vi "RoboDisplay7.vi"() -> ()   [LabVIEW 2013]
uses:
  GlobalPrevPage.vi
  GlobalPlotUpdateTime.vi
  GlobalSpeedUpdateTime.vi
  GlobalFavoriteNames.vi
  GlobalDisplayIndex.vi
  GlobalFavoritesList.vi
  GlobalRobotOffCheck.vi
  GlobalErrorCluster.vi
  GlobalErrorIndex.vi
  GlobalErrorCAN_ID.vi
  ErrorPrevValues.vi
  GlobalDataSize.vi
  GlobalSpeedArray.vi
  GlobalDataSelectArray.vi
  GlobalParamSize.vi
  GlobalFavorites.vi
  GlobalInitialParamVals.vi
  GlobalBatteryVoltageID.vi
  GlobalDataPath7.vi
  GlobalDataFileRefnum7.vi
  GlobalLabVIEWStart.vi
panel:
  out "MCU Elapsed mS 2":u32
  in  "Collect Data":bool
  out "Boolean":bool
  out "graph2labels":string[](array[string])
  out "graph1labels":string[](array[string])
  out "BATTERY VOLTAGE":dbl(knob) scale=20.0..30.0 scale format="%#_3g"
  in  "Tab Control":T1(tab)=enum."Display Data"
  out "Fav Error":bool[](array[boolean])
  in  "Remove":T2
  in  "Fav":T3
  in  "Commit":T4
  out "WAIT":bool
  in  "Reset default":bool
  out "Param #":dbl[](array[numeric])
  in  "Select 2":T5
  in  "Fav Input":dbl[](array[numeric])
  out "Value":dbl[](array[numeric])
  in  "Load":bool
  in  "Save":bool
  out "error":bool[](array[boolean])
  out "Param value":dbl[](array[numeric])
  out "Param #":dbl[](array[numeric])
  out "Param Name":string[](array[string])
  in  "Input":dbl[](array[numeric])
  in  "Page Select":dbl min=0.0 max=50.0 step=1.0
  out "Favorite Parameters":string[](array[string])
  in  "save data":bool
  in  "load data":bool
  out "Value 2":dbl[](array[numeric])
  out "Value 1":dbl[](array[numeric])
  out "Data # 2":dbl[](array[numeric])
  out "Data #":dbl[](array[numeric])
  out "Indicator":bool[](array[boolean])
  out "Array":string[](array[string])
  in  "Page":dbl min=0.0 max=50.0 step=1.0
  out "Number\nSelected":dbl
  out "Indicator 2":bool[](array[boolean])
  out "Array 2":string[](array[string])
  in  "Select":T3
  in  "?":T3
  out "Results":T6(array[cluster])
  in  "Search":string
  in  "Search \nButton":bool
  out "# of Results":i32
  in  "Speed Sel 2":enum32{"Slow", "Medium", "Fast"}[](array[radio])
  out "Speed 3":u32[](array[colorbox])
  out "Data Names 2":string[](array[string])
  out "Channel # 2":i16[](array[numeric])
  out "Data Value 2":sgl[](array[numeric]) format="%#_4g"
  out "Speed 2":u32[](array[colorbox])
  out "Data Names 1":string[](array[string])
  out "Channel # 1":i16[](array[numeric])
  out "Data Value 1":sgl[](array[numeric]) format="%#_4g"
  in  "One1":bool[](array[boolean])
  in  "One2":bool[](array[boolean])
  in  "Two1":bool[](array[boolean])
  in  "Two2":bool[](array[boolean])
  in  "Speed Sel":enum32{"Slow", "Medium", "Fast"}[](array[radio])
  in  "Clear Errors":bool
  in  "Pause Button":bool
  out "Error Description":string[](array[string])
  out "Board":string[](array[string])
  out "Error Name":string[](array[string])
  out "Freq.":dbl[](array[numeric])
  out "Time":dbl[](array[numeric])
  out "error message":bool
  out "Board Name 1":string
  out "Graph One":cluster{"Array":u32[], "Array 2":sgl[]}[](graph)
  in  "Graph\non":bool
  out "Error Name 1":string
  out "MCU Elapsed mS":u32 format="%<%H:%M:%S>t"
  in  "stop":bool
  out "Graph Two":cluster{"Array":u32[], "Array 2":sgl[]}[](graph)
  # "Robot Time:"
  # "ms timer:"
  # "DATA COLLECTION"
  # "Board"
  # "OFF"
  # "ON"
  # "Error Name"
  # "RoboDAQ\n\n(Version 7)\n\n\n\n\n\n\nCreated by: John Buzzi, Jason Cortell, Katie Hartl, Carlos Arango\n\nFall 2009"
  # "PLEASE LOOK AT SUGGESTIONS\nTAB IF YOU HAVE HELPFUL \nCOMMENTS!!"
  # "Favorites"
  # "Press [Home] to increment\nPress [End] to decrement"
  # "Press [Page Up] to increment\nPress [Page Down] to decrement"
  # "Select"
  # "Select"
  # "MAX ALLOWED: 48"
  # "NOT WORKING YET\n.\n.\n.\n.\n.\n.\n.\n......................."
  # "CAN ID"
  # "Name"
  # "Search Field"
  # "Note: Add function does not work yet"
  # "# of hits"
  # "Graphs"
  # "Graphs"
  # "Speed\n(S)   (M)   (F)"
  # "Speed\n(S)   (M)   (F)"
  # "Speed"
  # "Speed"
  # "Channel Name"
  # "One"
  # "Two"
  # "Channel Name"
  # "One"
  # "Two"
  # "SUGGESTIONS (double click text box to edit)\n\nMy to do list:\nFix error handling so that it works in the more advanced way that I had intended\nFix bug with speed select when data is de-selected and speeds are incorrect\nradio buttons\nload save data\nadd data by number\nmake index bigger\nslow default speed\n\n\nOther Suggestions/Comments (please add user input so that I can make the program better)\n- (nac) Change default folder for can_id.h and error_id.h to the Ranger Configuration folder\n\n\n\n\nNote: Strikeout = fixed"
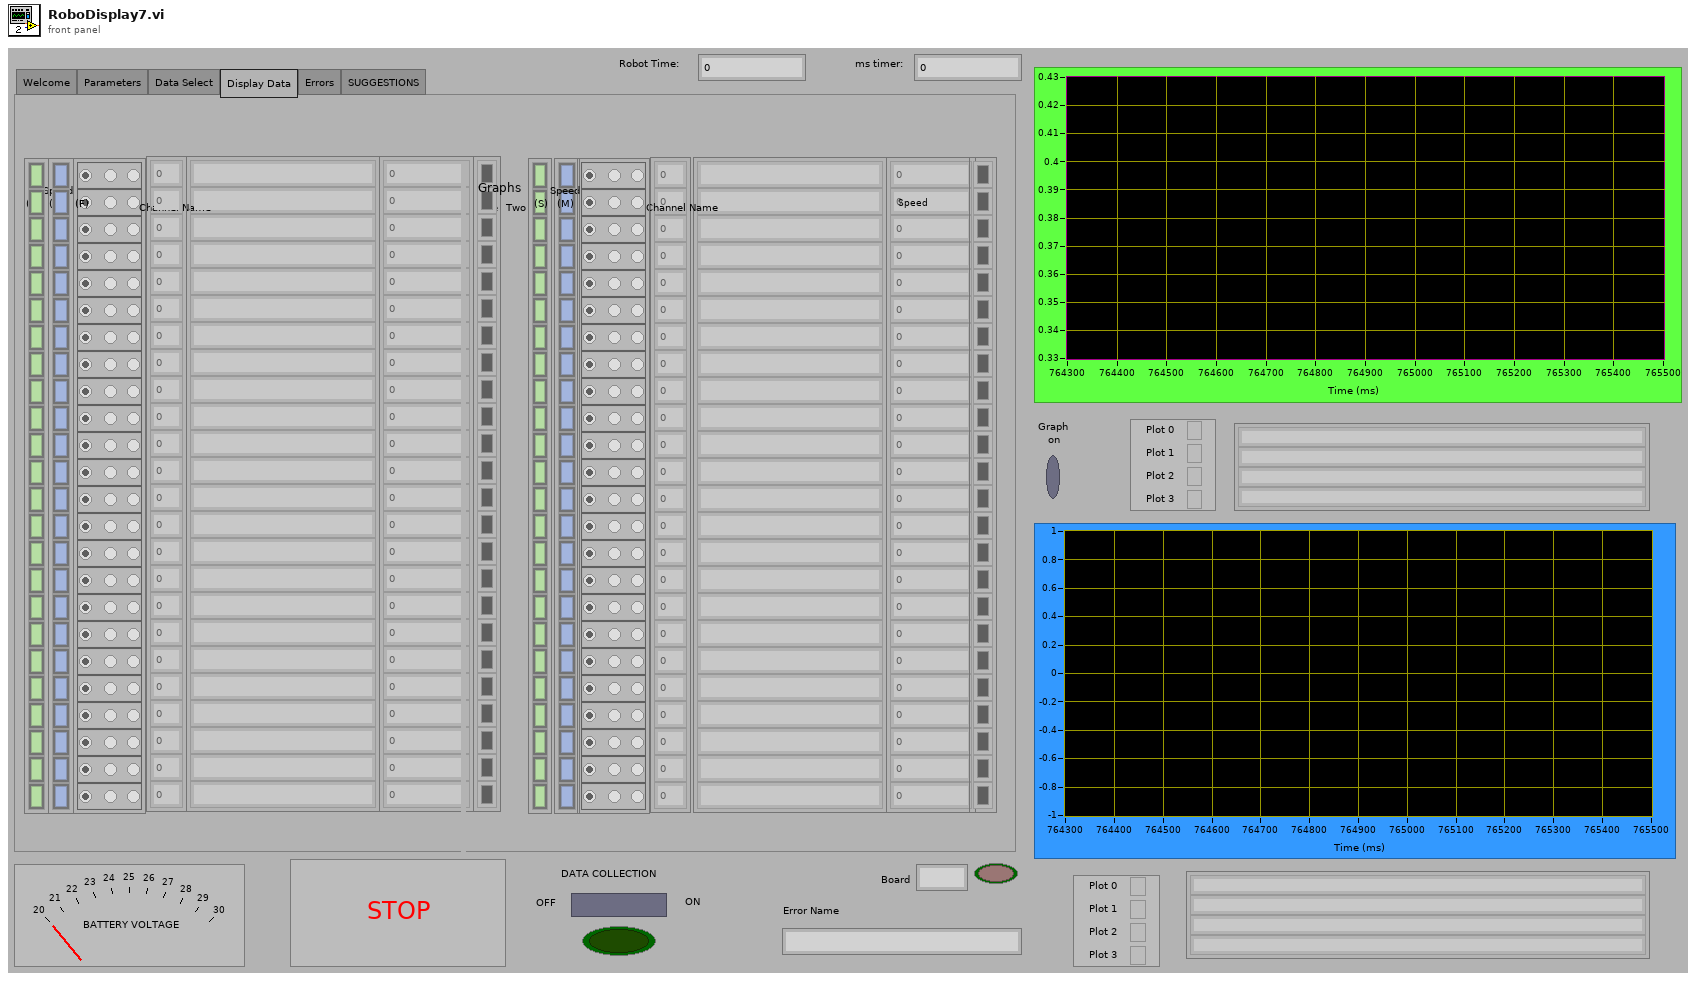
[diagram p1: front panel]
types:
  T1 = enum32{"Welcome", "Parameters", "Data Select", "Display Data", "Errors", "SUGGESTIONS"}
  T2 = cluster{"X button":bool, "X button 2":bool, "X button 3":bool, "X button 4":bool, "X button 5":bool, "X button 6":bool, "X button 7":bool, "X button 8":bool, "X button 9":bool, "X button 10":bool, "X button 11":bool, "X button 12":bool, "X button 13":bool, "X button 14":bool, "X button 15":bool, "X button 16":bool, "X button 17":bool, "X button 18":bool, "X button 19":bool, "X button 20":bool}
  T3 = cluster{"Boolean 2":bool, "Boolean 3":bool, "Boolean 4":bool, "Boolean 5":bool, "Boolean 6":bool, "Boolean 7":bool, "Boolean 8":bool, "Boolean 9":bool, "Boolean 10":bool, "Boolean 11":bool, "Boolean 12":bool, "Boolean 13":bool, "Boolean 14":bool, "Boolean 15":bool, "Boolean 16":bool, "Boolean 17":bool, "Boolean 18":bool, "Boolean 19":bool, "Boolean 20":bool, "Boolean 21":bool, "Boolean 22":bool, "Boolean 23":bool, "Boolean 24":bool, "Boolean 25":bool}
  T4 = cluster{"Boolean":bool, "Boolean 2":bool, "Boolean 3":bool, "Boolean 4":bool, "Boolean 5":bool, "Boolean 6":bool, "Boolean 7":bool, "Boolean 8":bool, "Boolean 9":bool, "Boolean 10":bool, "Boolean 11":bool, "Boolean 12":bool, "Boolean 13":bool, "Boolean 14":bool, "Boolean 15":bool, "Boolean 16":bool, "Boolean 17":bool, "Boolean 18":bool, "Boolean 19":bool, "Boolean 20":bool}
  T5 = cluster{"Boolean":bool, "Boolean 2":bool, "Boolean 3":bool, "Boolean 4":bool, "Boolean 5":bool, "Boolean 6":bool, "Boolean 7":bool, "Boolean 8":bool, "Boolean 9":bool, "Boolean 10":bool, "Boolean 11":bool, "Boolean 12":bool, "Boolean 13":bool, "Boolean 14":bool, "Boolean 15":bool, "Boolean 16":bool, "Boolean 17":bool, "Boolean 18":bool, "Boolean 19":bool, "Boolean 20":bool, "Boolean 21":bool, "Boolean 22":bool, "Boolean 23":bool, "Boolean 24":bool}
  T6 = cluster{"Result Index":dbl, "Results 3":string, "Boolean 2":bool}[]
  T7 = cluster{"Error ID":i32, "Board ID":i32, "Time":u32, "Frequency":i32}[]
  T8 = enum16{"open", "replace", "create", "open or create", "replace or create", "replace or create with confirmation"}
  T9 = cluster{"Numeric":dbl, "String":string, "ignore case? (F)":bool}
  T10 = cluster{"Numeric":dbl, "String":string, "ignore case? (F)":bool}[]
  T11 = cluster{"Frequency":dbl, "Description":string, "Error Name":string, "Board Name":string, " Board Source":dbl, "Timestamp":dbl}[]
  T12 = cluster{"Frequency":dbl, "Description":string, "Error Name":string, "Board Name":string, " Board Source":dbl, "Timestamp":dbl}
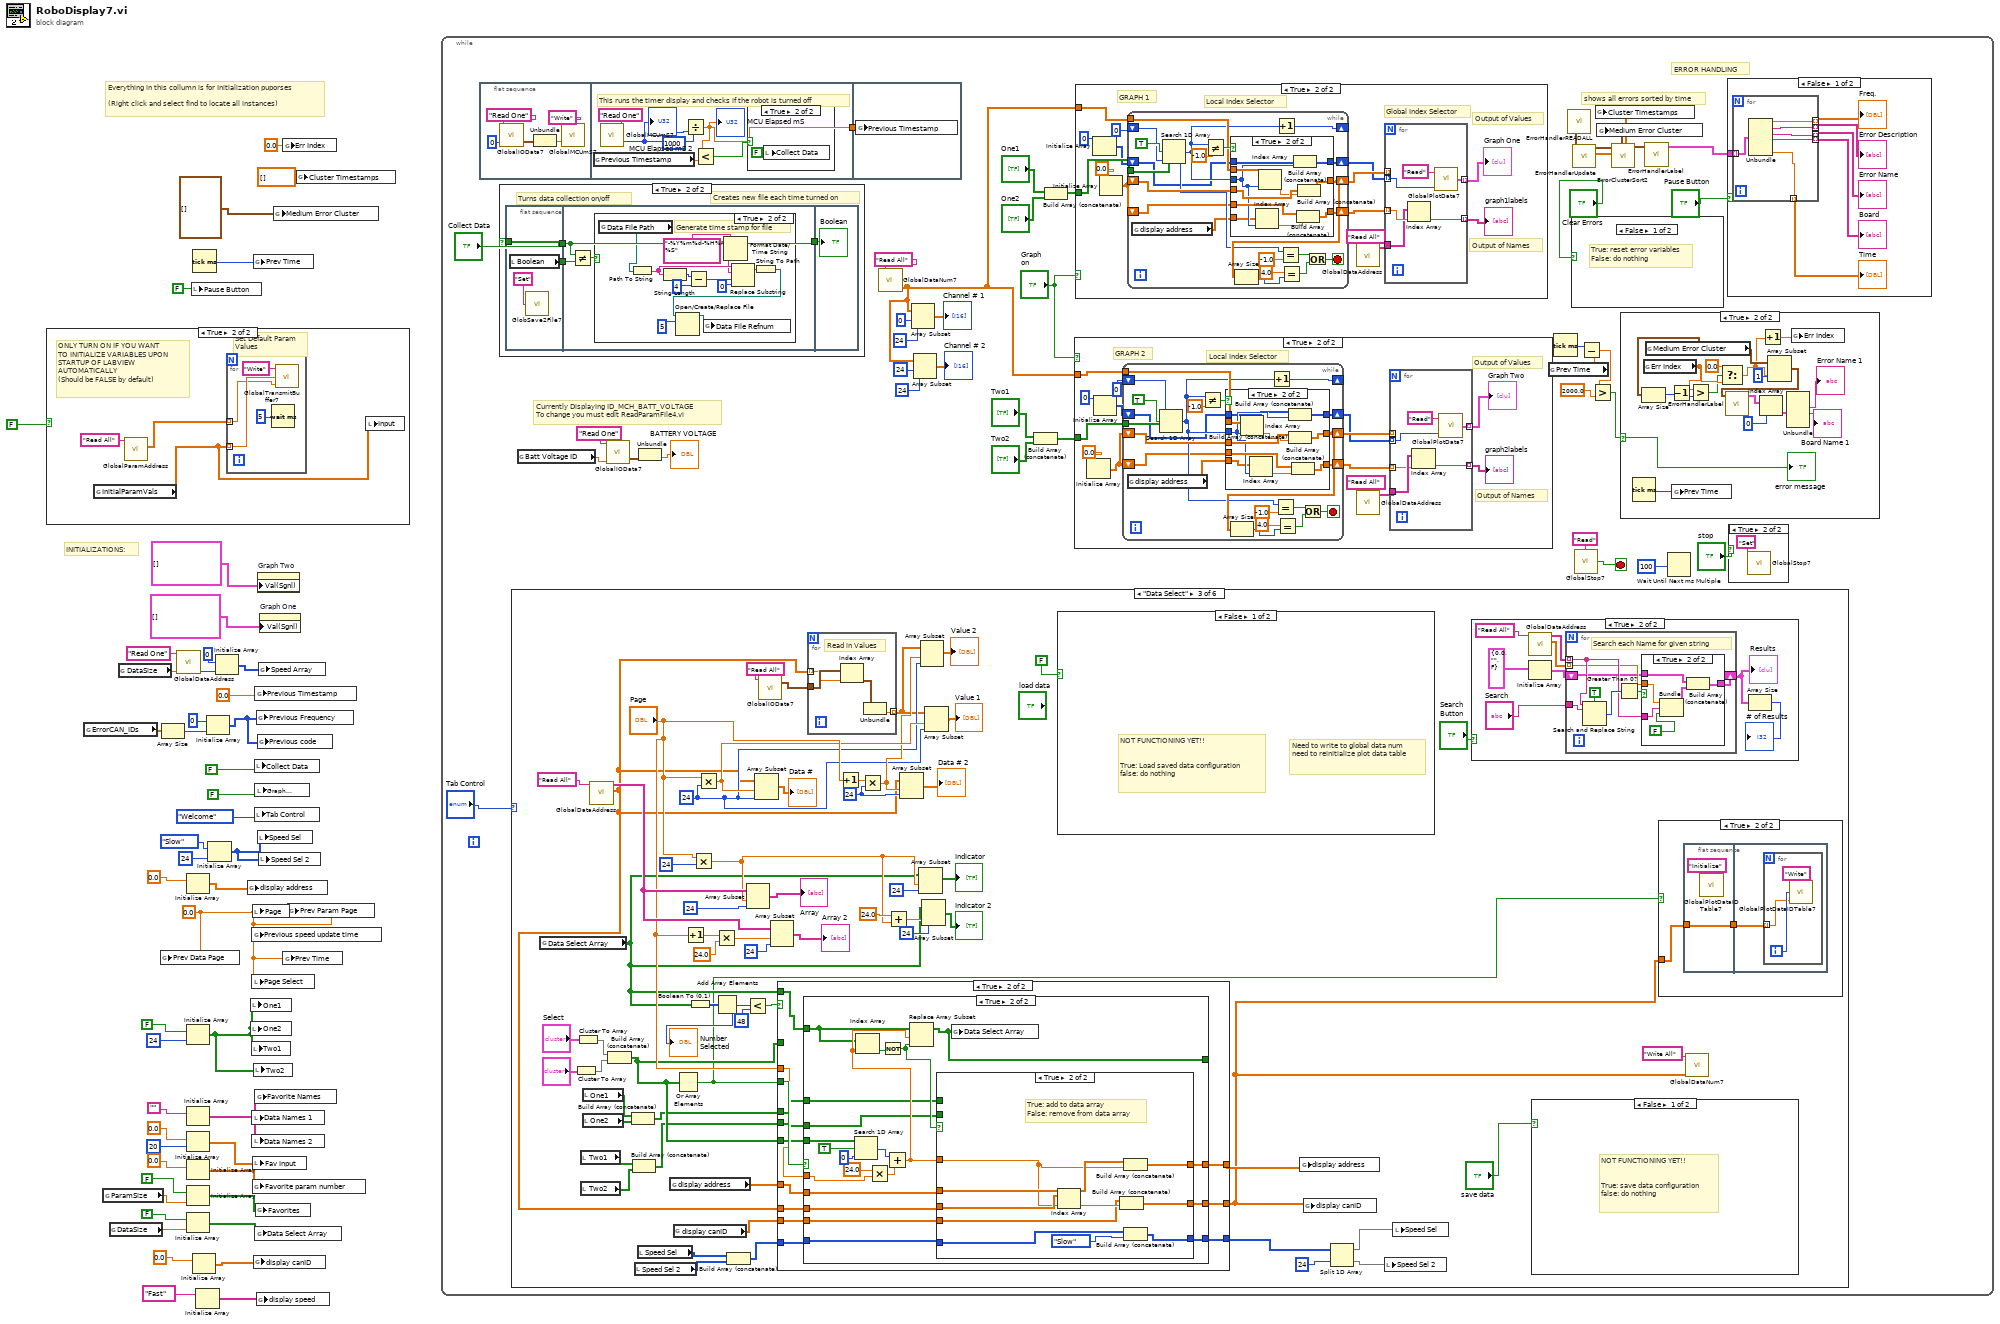
[diagram p0: block diagram]
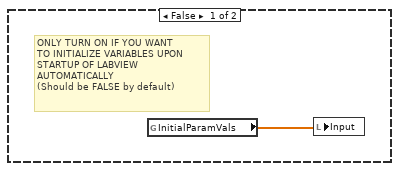
[diagram p2: hidden frame]
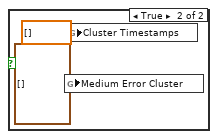
[diagram p3: hidden frame]
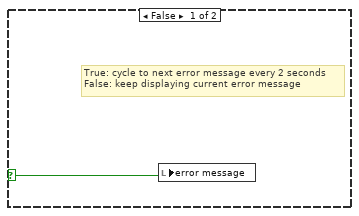
[diagram p4: hidden frame]
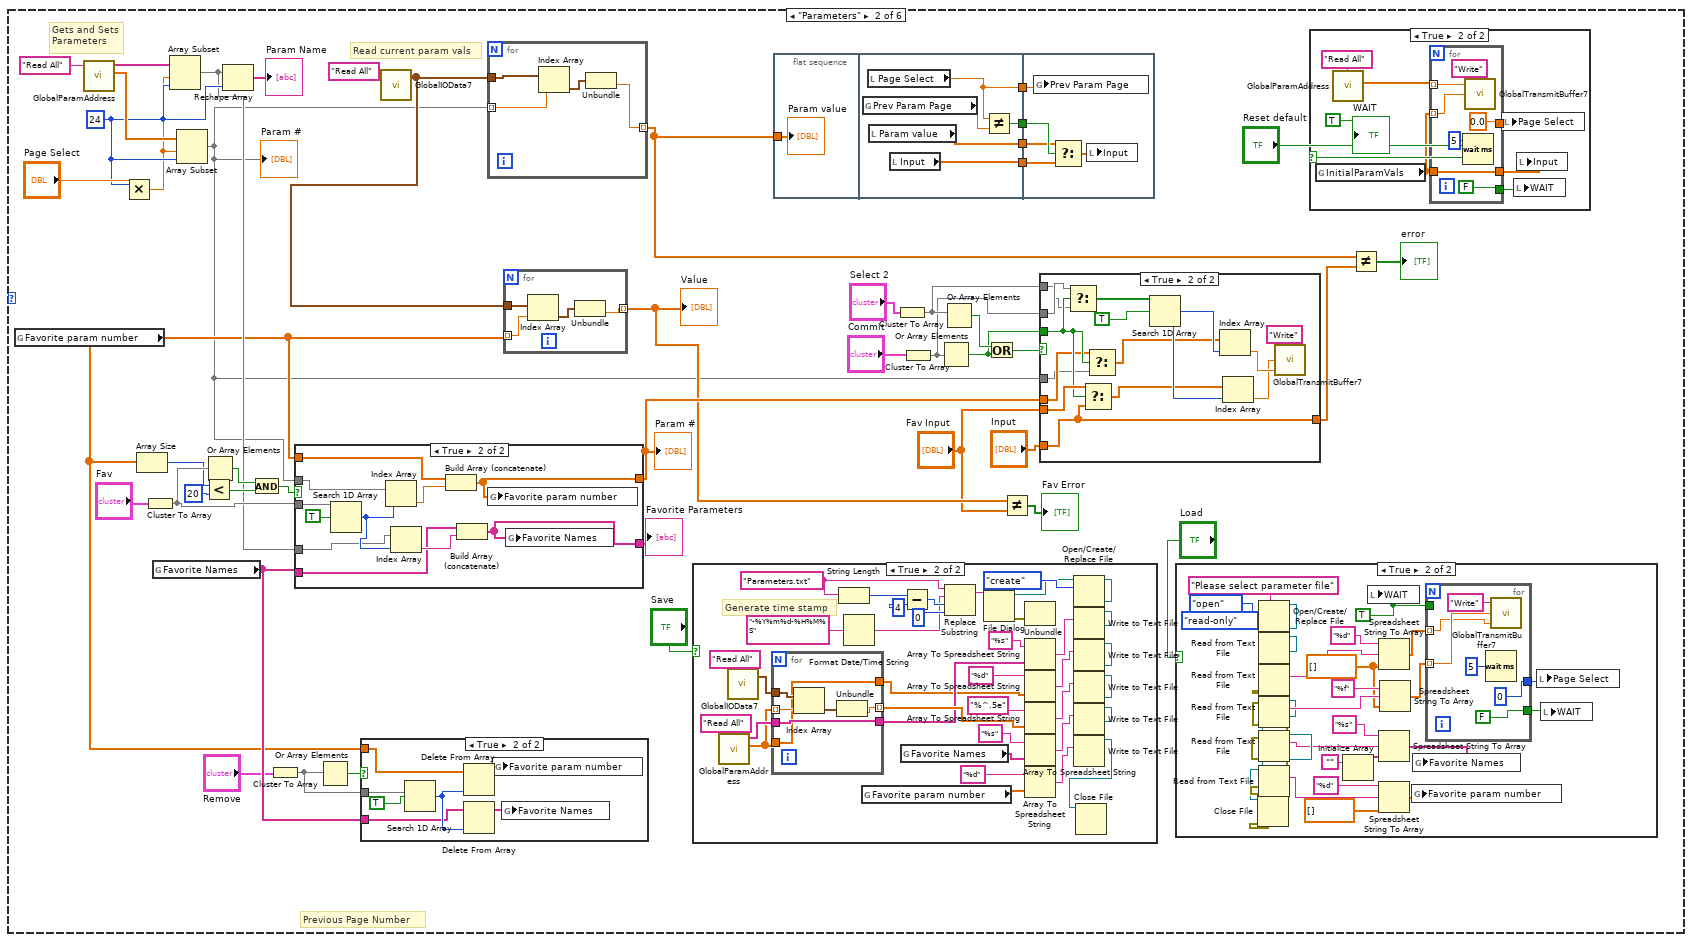
[diagram p12: hidden frame]
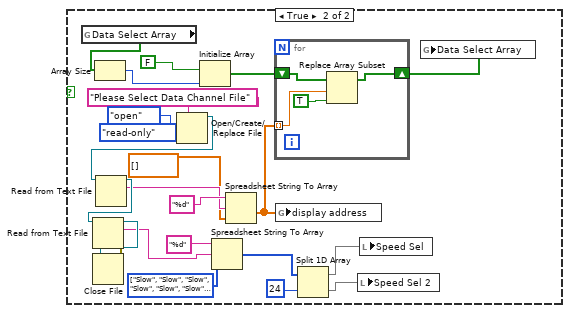
[diagram p19: hidden frame]
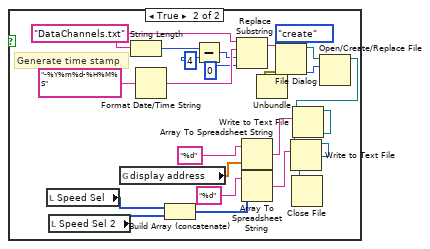
[diagram p20: hidden frame]
diagram:
  w13 = 0.0 ("Previous speed update time")
  # "Everything in this collumn is for Initialization puporses\n\n(Right click and select find to locate all instances)"
  # "INITIALIZATIONS:"
  n1 = case shown="True" FALSE {
    frame False {
      # "ONLY TURN ON IF YOU WANT\nTO INITIALIZE VARIABLES UPON\nSTARTUP OF LABVIEW \nAUTOMATICALLY \n(Should be FALSE by default)"
      n2 = global read "GlobalInitialParamVals.vi" "InitialParamVals"() -> (w48:dbl[])
      n3 = local write "Input"(w48) -> ()
    }
    frame True {
      # "ONLY TURN ON IF YOU WANT\nTO INITIALIZE VARIABLES UPON\nSTARTUP OF LABVIEW \nAUTOMATICALLY \n(Should be FALSE by default)"
      # "Set Default Param\nValues"
      n4 = global read "GlobalInitialParamVals.vi" "InitialParamVals"() -> (w49:dbl[])
      n5 = call "GlobalParamAddress.vi"("Function select"="Read All") -> ("Parameter ID Out"=w51:dbl[])  [unwired: 3 in, 3 out]
      n6 = for {
        tunnel: w51 -> [w53] mode=indexing
        tunnel: w49 -> [w54] mode=indexing
        n7 = Wait (ms)(milliseconds to wait=u32 5) -> ()  [unwired: 1 out]
        n8 = call "GlobalTransmitBuffer7.vi"("Data_ID # in"=w53, "Value in"=w54, "Function select"="Write") -> ()  [unwired: 3 out]
      }
      n9 = local write "Input"(w49) -> ()
    }
  }
  n10 = global read "GlobalErrorCAN_ID.vi" "ErrorCAN_IDs"() -> (w42:dbl[])
  n11 = global read "GlobalParamSize.vi" "ParamSize"() -> (w25:dbl)
  n12 = global read "GlobalDataSize.vi" "DataSize"() -> (w30:dbl)
  n13 = global read "GlobalDataSize.vi" "DataSize"() -> (w34:dbl)
  n14 = global write "GlobalPrevPage.vi" "Prev Data Page"(w13) -> ()
  n15 = Array Size(array=w42) -> (size(s)=w40:i32)
  n16 = call "GlobalDataAddress.vi"("Element index"=w34, "Function select"="Read One") -> ("Data ID"=w33:u16)  [unwired: 2 in, 3 out]
  n17 = Initialize Array(0.0 ("Previous speed update time")) -> (w37:dbl[])  [unwired: 1 in]
  n18 = Initialize Array(FALSE ("Graph\non"), 24 ("dimension size")) -> (w23:bool[])
  n19 = Initialize Array("") -> (w19:string[])  [unwired: 1 in]
  n20 = Initialize Array(0.0 ("Previous speed update time"), 20 ("dimension size")) -> (w21:dbl[])
  n21 = Initialize Array(0.0 ("Previous speed update time")) -> (w27:dbl[])  [unwired: 1 in]
  n22 = Initialize Array(FALSE, w25) -> (w24:bool[])
  n23 = Initialize Array(FALSE, w30) -> (w28:bool[])
  n24 = local write "Pause Button"(FALSE ("Pause Button")) -> ()
  n25 = Initialize Array(0.0 ("Previous speed update time")) -> (w11:dbl[])  [unwired: 1 in]
  n26 = Tick Count (ms)() -> (millisecond timer value=w2:u32)
  n27 = Initialize Array("Fast" ("Combo Box")) -> (w9:string[])  [unwired: 1 in]
  n28 = Initialize Array(0 ("dimension size"), w40) -> (w39:i32[])
  n29 = Initialize Array(enum32{"Slow", "Medium", "Fast"}."Slow" ("Radio Buttons 2"), 24 ("dimension size")) -> (w3:enum32{"Slow", "Medium", "Fast"}[])
  n30 = Initialize Array(0, w33) -> (w31:i32[])
  n31 = global write "GlobalDisplayIndex.vi" "display address"(w37) -> ()
  n32 = local write "One1"(w23) -> ()
  n33 = local write "One2"(w23) -> ()
  n34 = local write "Two1"(w23) -> ()
  n35 = global write "GlobalSpeedUpdateTime.vi" "Previous speed update time"(w13) -> ()
  n36 = local write "Page Select"(w13) -> ()
  n37 = local write "Data Names 1"(w19) -> ()
  n38 = local write "Data Names 2"(w19) -> ()
  n39 = local write "Page"(w13) -> ()
  n40 = local write "Fav Input"(w21) -> ()
  n41 = global write "GlobalFavoritesList.vi" "Favorite param number"(w27) -> ()
  n42 = global write "GlobalPlotUpdateTime.vi" "Prev Time"(w2) -> ()
  n43 = local write "Two2"(w23) -> ()
  n44 = global write "GlobalDisplayIndex.vi" "display canID"(w11) -> ()
  n45 = local write "Collect Data"(FALSE ("Boolean 2")) -> ()
  n46 = local write "Tab Control"(T1."Welcome" ("Tab Control")) -> ()
  n47 = global write "GlobalRobotOffCheck.vi" "Previous Timestamp"(0.0 ("Previous Timestamp")) -> ()
  n48 = local write "Graph\non"(FALSE ("Graph\non")) -> ()
  n49 = global write "GlobalFavoriteNames.vi" "Favorite Names"(w19) -> ()
  n50 = global write "GlobalDataSelectArray.vi" "Data Select Array"(w28) -> ()
  n51 = global write "GlobalFavorites.vi" "Favorites"(w24) -> ()
  n52 = global write "ErrorPrevValues.vi" "Previous Frequency"(w39) -> ()
  n53 = global write "GlobalDisplayIndex.vi" "display speed"(w9) -> ()
  n54 = global write "ErrorPrevValues.vi" "Previous code"(w39) -> ()
  n55 = local write "Speed Sel"(w3) -> ()
  n56 = property on="Graph Two" class="XYGraph (strict)"("Val(Sgnl)"=cluster{"Array":dbl[], "Array 2":dbl[]}[] [] ("Value (Signaling)")) -> ()  [unwired: 2 in, 2 out]
  n57 = global write "GlobalSpeedArray.vi" "Speed Array"(w31) -> ()
  n58 = local write "Speed Sel 2"(w3) -> ()
  n59 = property on="Graph One" class="XYGraph (strict)"("Val(Sgnl)"=cluster{"Array":dbl[], "Array 2":dbl[]}[] [] ("Value (Signaling)")) -> ()  [unwired: 2 in, 2 out]
  n60 = global write "GlobalErrorCluster.vi" "Medium Error Cluster"(T7 [] ("Medium Error Cluster")) -> ()
  n61 = global write "GlobalErrorIndex.vi" "Err Index"(0.0 ("Err Index")) -> ()
  n62 = global write "GlobalPlotUpdateTime.vi" "Prev Time"(w13) -> ()
  n63 = global write "GlobalPrevPage.vi" "Prev Param Page"(w13) -> ()
  n64 = global write "GlobalErrorCluster.vi" "Cluster Timestamps"(dbl[] [] ("Cluster Timestamps")) -> ()
  n65 = while {
    stop <- w91 stop-if-true
    # "shows all errors sorted by time"
    # "Currently Displaying ID_MCH_BATT_VOLTAGE\nTo change you must edit ReadParamFile4.vi"
    # "ERROR HANDLING"
    n66 = flat-sequence {
      tunnel: [w133] -> w73
      tunnel: w73 -> [w139]
      frame #0 {
        n67 = call "GlobalIOData7.vi"("Function select"="Read One", "IO Data ID"=u32 0) -> ("IO data out"=w129:cluster{"Time":u32, "Value":sgl})  [unwired: 3 in, 1 out]
        n68 = Unbundle(w129) -> ("Value"=w128:sgl)  [unwired: 1 out]
        n69 = call "GlobalMCUmS7.vi"("mS In"=w128, "Function select"="Write") -> ()  [unwired: 2 out]
      }
      frame #1 {
        # "This runs the timer display and checks if the robot is turned off"
        n70 = global read "GlobalRobotOffCheck.vi" "Previous Timestamp"() -> (w135:dbl)
        n71 = call "GlobalMCUmS7.vi"("Function select"="Read One") -> ("mS Out"=w132:u32)  [unwired: 1 in, 1 out]
        "MCU Elapsed mS 2" <- w132
        n72 = Divide(x=w132, y=u32 1000) -> (x/y=w133:dbl)
        "MCU Elapsed mS" <- w133
        n73 = Less?(x=w133, y=w135) -> (x < y?=w136:bool)
        n74 = case shown="True" w136 {
          frame False {
          }
          frame True {
            n75 = local write "Collect Data"(FALSE ("Collect Data")) -> ()
          }
        }
      }
      frame #2 {
        n76 = global write "GlobalRobotOffCheck.vi" "Previous Timestamp"(w139) -> ()
      }
    }
    n77 = case shown="True" "Collect Data" {
      selector: "Collect Data" -> [w783 w788]
      frame False {
        # "True: data collection on\nFalse: data collection off"
        n78 = call "GlobSave2File7.vi"("Function select"="Clear") -> ()  [unwired: 1 out]
        n79 = local write "Boolean"(w783) -> ()
      }
      frame True {
        # "Creates new file each time turned on"
        # "Turns data collection on/off"
        n80 = flat-sequence {
          tunnel: w788 -> [w790]
          tunnel: [w790] -> w787
          tunnel: [w789] -> w785
          tunnel: w787 -> [w793]
          tunnel: [w793] -> w786
          tunnel: w785 -> [w792]
          tunnel: w786 -> [w807]
          frame #0 {
            n81 = local read "Boolean"() -> (w789:bool)
            n82 = call "GlobSave2File7.vi"("Function select"="Set") -> ()  [unwired: 1 out]
          }
          frame #1 {
            n83 = Not Equal?(x=w793, y=w792) -> (x != y?=w794:bool)
            n84 = case shown="True" w794 {
              frame False {
              }
              frame True {
                # "Generate time stamp for file"
                n85 = global read "GlobalDataPath7.vi" "Data File Path"() -> (w795:path)
                n86 = Path To String(path=w795) -> (string=w805:string)
                n87 = String Length(string=w805) -> (length=w798:i32)
                n88 = Subtract(x=w798, y=4) -> (x-y=w800:i32)
                n89 = Format Date/Time String(time format string (%c)="-%Y%m%d-%H%M%S") -> (date/time string=w804:string)  [unwired: 2 in]
                n90 = Replace Substring(2:0, 3:w800, 4:w804, 5:w805) -> (1:w802:string)  [unwired: 1 out]
                n91 = String To Path(string=w802) -> (path=w806:path)
                n92 = Open/Create/Replace File(file path (use dialog)=w806, operation (0:open)=5) -> (refnum out=w797:refnum<file>)  [unwired: 4 in, 2 out]
                n93 = global write "GlobalDataFileRefnum7.vi" "Data File Refnum"(w797) -> ()
              }
            }
          }
          frame #2 {
            "Boolean" <- w807
          }
        }
      }
    }
    n94 = case shown="\"Data Select\"" "Tab Control" {
      frame "Welcome", Default {
        # "Introduction Page"
      }
      frame "Parameters" {
        w277 = 24 ("index")
        # "Read current param vals"
        # "Previous Page Number"
        # "Gets and Sets\nParameters"
        n95 = global read "GlobalFavoritesList.vi" "Favorite param number"() -> (w262:dbl[])
        n96 = call "GlobalParamAddress.vi"("Function select"="Read All") -> ("Parameter ID Out"=w290:dbl[], "Parameter Names Out"=w289:string[])  [unwired: 3 in, 2 out]
        n97 = Multiply(x=w277, y="Page Select") -> (x*y=w276:dbl)
        n98 = Array Size(array=w262) -> (size(s)=w273:i32)
        n99 = Cluster To Array(cluster="Fav") -> (array=w274:bool[])
        n100 = global read "GlobalFavoriteNames.vi" "Favorite Names"() -> (w263:string[])
        n101 = Array Subset(array=w289, index=w276, length=w277) -> (w266:string[])
        n102 = Array Subset(array=w290, index=w276, length=w277) -> (w250:dbl[])
        "Param #" <- w250
        n103 = Less?(x=w273, y=20) -> (x < y?=w269:bool)
        n104 = Or Array Elements(Boolean array=w274) -> (logical OR=w270:bool)
        n105 = Reshape Array(w266, w277) -> (→"Param Name":string[])
        n106 = And(x=w270, y=w269) -> (x .and. y?=w271:bool)
        n107 = Cluster To Array(cluster="Remove") -> (array=w260:bool[])
        n108 = case shown="True" w271 {
          tunnel: w250 -> [_ w330]
          tunnel: w274 -> [_ w328]
          tunnel: w262 -> [w319 w326]
          tunnel: [w319 w325] -> w268
          tunnel: w263 -> [w318 w323]
          tunnel: w266 -> [_ w321]
          tunnel: [w318 w320] -> w265
          frame False {
            # "True: Add a favorite\nFalse: Do nothing"
          }
          frame True {
            n109 = Search 1D Array(1D array=w328, element=TRUE) -> (index of element=w322:i32)  [unwired: 1 in]
            n110 = Index Array(array=w330, index=w322) -> (element=w329:dbl)
            n111 = Index Array(array=w321, index=w322) -> (element=w324:string)
            n112 = Build Array (concatenate)(w326, w329) -> (w325:dbl[])
            n113 = Build Array (concatenate)(w323, w324) -> (w320:string[])
            n114 = global write "GlobalFavoritesList.vi" "Favorite param number"(w325) -> ()
            n115 = global write "GlobalFavoriteNames.vi" "Favorite Names"(w320) -> ()
          }
        }
        "Param #" <- w268
        "Favorite Parameters" <- w265
        n116 = Or Array Elements(Boolean array=w260) -> (logical OR=w264:bool)
        n117 = case shown="True" w264 {
          tunnel: w260 -> [_ w312]
          tunnel: w263 -> [_ w308]
          tunnel: w262 -> [_ w310]
          frame False {
            # "True: Remove a favorite\nFalse: do nothing"
          }
          frame True {
            n118 = Search 1D Array(1D array=w312, element=TRUE) -> (index of element=w311:i32)  [unwired: 1 in]
            n119 = Delete From Array(array=w310, index=w311) -> (array with subset deleted=w309:dbl[])  [unwired: 1 in, 1 out]
            n120 = Delete From Array(array=w308, index=w311) -> (array with subset deleted=w307:string[])  [unwired: 1 in, 1 out]
            n121 = global write "GlobalFavoritesList.vi" "Favorite param number"(w309) -> ()
            n122 = global write "GlobalFavoriteNames.vi" "Favorite Names"(w307) -> ()
          }
        }
        n123 = call "GlobalIOData7.vi"("Function select"="Read All") -> ("Array"=w267:cluster{"Time":u32, "Value":sgl}[])  [unwired: 4 in, 1 out]
        n124 = for {
          tunnel: w250 -> [w392] mode=indexing
          tunnel: w267 -> [w391]
          tunnel: [w389] -> w251 mode=indexing
          n125 = Index Array(array=w391, index=w392) -> (element=w390:cluster{"Time":u32, "Value":sgl})
          n126 = Unbundle(w390) -> ("Value"=w389:sgl)  [unwired: 1 out]
        }
        n127 = for {
          tunnel: w262 -> [w317] mode=indexing
          tunnel: w267 -> [w316]
          tunnel: [w314] -> w259 mode=indexing
          n128 = Index Array(array=w316, index=w317) -> (element=w315:cluster{"Time":u32, "Value":sgl})
          n129 = Unbundle(w315) -> ("Value"=w314:sgl)  [unwired: 1 out]
        }
        "Value" <- w259
        n130 = case shown="True" "Save" {
          frame False {
            # "True: Save parameters and favorites\nFalse: do nothing"
          }
          frame True {
            w352 = "Parameters.txt" ("Default file name")
            # "Generate time stamp"
            n131 = call "GlobalParamAddress.vi"("Function select"="Read All") -> ("Parameter ID Out"=w347:dbl[], "Parameter Names Out"=w366:string[])  [unwired: 3 in, 2 out]
            n132 = call "GlobalIOData7.vi"("Function select"="Read All") -> ("Array"=w364:cluster{"Time":u32, "Value":sgl}[])  [unwired: 4 in, 1 out]
            n133 = for {
              tunnel: w366 -> [w370]
              tunnel: w347 -> [w374] mode=indexing
              tunnel: w364 -> [w373]
              tunnel: [w371] -> w363 mode=indexing
              tunnel: [w370] -> w361
              tunnel: w347 -> [w369]
              tunnel: [w369] -> w342
              n134 = Index Array(array=w373, index=w374) -> (element=w372:cluster{"Time":u32, "Value":sgl})
              n135 = Unbundle(w372) -> ("Value"=w371:sgl)  [unwired: 1 out]
            }
            n136 = String Length(string=w352) -> (length=w354:i32)
            n137 = Format Date/Time String(time format string (%c)="-%Y%m%d-%H%M%S") -> (date/time string=w348:string)  [unwired: 2 in]
            n138 = global read "GlobalFavoritesList.vi" "Favorite param number"() -> (w335:dbl[])
            n139 = global read "GlobalFavoriteNames.vi" "Favorite Names"() -> (w336:string[])
            n140 = Subtract(x=w354, y=4) -> (x-y=w350:i32)
            n141 = Replace Substring(2:0, 3:w350, 4:w348, 5:w352) -> (1:w353:string)  [unwired: 1 out]
            n142 = File Dialog(9:w353) -> (0:w356:errorcluster, 3:w355:path)  [unwired: 6 in, 2 out]
            n143 = Unbundle(w356) -> ()  [unwired: 3 out]
            n144 = Array To Spreadsheet String(array=w361, 3:"%s") -> (spreadsheet string=w358:string)  [unwired: 1 in]
            n145 = Array To Spreadsheet String(array=w342, 3:"%d") -> (spreadsheet string=w343:string)  [unwired: 1 in]
            n146 = Array To Spreadsheet String(array=w363, 3:"%^.5e") -> (spreadsheet string=w341:string)  [unwired: 1 in]
            n147 = Array To Spreadsheet String(array=w336, 3:"%s") -> (spreadsheet string=w338:string)  [unwired: 1 in]
            n148 = Array To Spreadsheet String(array=w335, 3:"%d") -> (spreadsheet string=w337:string)  [unwired: 1 in]
            n149 = Open/Create/Replace File(file path (use dialog)=w355, operation (0:open)=T8."create") -> (refnum out=w357:refnum<file>, error out=w332:errorcluster)  [unwired: 4 in, 1 out]
            n150 = Write to Text File(file (use dialog)=w357, text=w358, error in=w332) -> (refnum out=w346:refnum<file>)  [unwired: 1 in, 2 out]
            n151 = Write to Text File(file (use dialog)=w346, text=w343) -> (refnum out=w345:refnum<file>)  [unwired: 2 in, 2 out]
            n152 = Write to Text File(file (use dialog)=w345, text=w341) -> (refnum out=w340:refnum<file>)  [unwired: 2 in, 2 out]
            n153 = Write to Text File(file (use dialog)=w340, text=w338) -> (refnum out=w339:refnum<file>)  [unwired: 2 in, 2 out]
            n154 = Write to Text File(file (use dialog)=w339, text=w337) -> (refnum out=w331:refnum<file>)  [unwired: 2 in, 2 out]
            n155 = Close File(refnum=w331) -> ()  [unwired: 1 in, 2 out]
          }
        }
        n156 = flat-sequence {
          tunnel: w251 -> [w296]
          tunnel: [w300] -> w256
          tunnel: [w299] -> w255
          tunnel: [w298] -> w253
          tunnel: [w297] -> w252
          tunnel: w256 -> [w306]
          tunnel: w255 -> [w304]
          tunnel: w252 -> [w303]
          tunnel: w253 -> [w302]
          frame #0 {
            "Param value" <- w296
          }
          frame #1 {
            n157 = global read "GlobalPrevPage.vi" "Prev Param Page"() -> (w301:dbl)
            n158 = local read "Page Select"() -> (w300:dbl)
            n159 = local read "Param value"() -> (w297:dbl[])
            n160 = local read "Input"() -> (w298:dbl[])
            n161 = Not Equal?(x=w300, y=w301) -> (x != y?=w299:bool)
          }
          frame #2 {
            n162 = global write "GlobalPrevPage.vi" "Prev Param Page"(w306) -> ()
            n163 = Select(t=w303, s=w304, f=w302) -> (s? t:f=w305:dbl[])
            n164 = local write "Input"(w305) -> ()
          }
        }
        n165 = Cluster To Array(cluster="Select 2") -> (array=w285:bool[])
        n166 = Cluster To Array(cluster="Commit") -> (array=w278:bool[])
        n167 = Or Array Elements(Boolean array=w278) -> (logical OR=w279:bool)
        n168 = Or Array Elements(Boolean array=w285) -> (logical OR=w281:bool)
        n169 = Or(x=w281, y=w279) -> (x .or. y?=w280:bool)
        n170 = Not Equal?(x=w259, y="Fav Input") -> (x != y?=→"Fav Error":bool[])
        n171 = case shown="True" w280 {
          tunnel: w285 -> [_ w394]
          tunnel: "Input" -> [w393 w402]
          tunnel: [w393 w402] -> w292
          tunnel: w250 -> [_ w396]
          tunnel: w279 -> [_ w399]
          tunnel: "Fav Input" -> [_ w401]
          tunnel: w278 -> [_ w395]
          tunnel: w268 -> [_ w397]
          frame False {
            # "True: commit selected parameter value to the\ntransmit buffer \n\nFalse: do nothing"
          }
          frame True {
            n172 = Select(t=w395, s=w399, f=w394) -> (s? t:f=w400:bool[])
            n173 = Select(t=w401, s=w399, f=w402) -> (s? t:f=w403:dbl[])
            n174 = Select(t=w397, s=w399, f=w396) -> (s? t:f=w398:dbl[])
            n175 = Search 1D Array(1D array=w400, element=TRUE) -> (index of element=w407:i32)  [unwired: 1 in]
            n176 = Index Array(array=w398, index=w407) -> (element=w406:dbl)
            n177 = Index Array(array=w403, index=w407) -> (element=w405:dbl)
            n178 = call "GlobalTransmitBuffer7.vi"("Data_ID # in"=w406, "Value in"=w405, "Function select"="Write") -> ()  [unwired: 3 out]
          }
        }
        n179 = case shown="True" "Load" {
          frame False {
            # "True: Load saved parameters and favorites\nFalse: Do nothing"
          }
          frame True {
            w428 = sgl[] []
            w426 = TRUE ("Wait")
            n180 = Open/Create/Replace File(prompt="Please select parameter file", operation (0:open)=T8."open", access (0:read/write)=enum16{"read/write", "read-only", "write-only"}."read-only") -> (refnum out=w439:refnum<file>)  [unwired: 3 in, 2 out]
            n181 = Read from Text File(file (use dialog)=w439) -> (refnum out=w437:refnum<file>, error out=w438:errorcluster)  [unwired: 3 in, 2 out]
            n182 = Read from Text File(file (use dialog)=w437, error in=w438) -> (refnum out=w435:refnum<file>, text=w434:string, error out=w436:errorcluster)  [unwired: 2 in, 1 out]
            n183 = Read from Text File(file (use dialog)=w435, error in=w436) -> (refnum out=w422:refnum<file>, text=w432:string, error out=w423:errorcluster)  [unwired: 2 in, 1 out]
            n184 = Read from Text File(file (use dialog)=w422, error in=w423) -> (refnum out=w420:refnum<file>, text=w419:string, error out=w421:errorcluster)  [unwired: 2 in, 1 out]
            n185 = Read from Text File(file (use dialog)=w420, error in=w421) -> (refnum out=w409:refnum<file>, text=w416:string, error out=w410:errorcluster)  [unwired: 2 in, 1 out]
            n186 = Close File(refnum=w409, error in=w410) -> ()  [unwired: 2 out]
            n187 = Initialize Array("") -> (w413:string[])  [unwired: 1 in]
            n188 = local write "WAIT"(w426) -> ()
            n189 = Spreadsheet String To Array(format string="%d", spreadsheet string=w434, array type (2D Dbl)=w428) -> (array=w433:sgl[])  [unwired: 1 in]
            n190 = Spreadsheet String To Array(format string="%s", spreadsheet string=w419, array type (2D Dbl)=w413) -> (array=w412:string[])  [unwired: 1 in]
            n191 = Spreadsheet String To Array(format string="%d", spreadsheet string=w416, array type (2D Dbl)=sgl[] []) -> (array=w417:sgl[])  [unwired: 1 in]
            n192 = Spreadsheet String To Array(format string="%f", spreadsheet string=w432, array type (2D Dbl)=w428) -> (array=w429:sgl[])  [unwired: 1 in]
            n193 = global write "GlobalFavoritesList.vi" "Favorite param number"(w417) -> ()
            n194 = global write "GlobalFavoriteNames.vi" "Favorite Names"(w412) -> ()
            n195 = for {
              tunnel: w433 -> [w445] mode=indexing
              tunnel: w429 -> [w446] mode=indexing
              tunnel: [FALSE ("Wait")] -> w441
              tunnel: [0] -> w427
              tunnel: w426 -> [_]
              n196 = Wait (ms)(milliseconds to wait=u32 5) -> ()  [unwired: 1 out]
              n197 = call "GlobalTransmitBuffer7.vi"("Data_ID # in"=w445, "Value in"=w446, "Function select"="Write") -> ()  [unwired: 3 out]
            }
            n198 = local write "Page Select"(w427) -> ()
            n199 = local write "WAIT"(w441) -> ()
          }
        }
        n200 = case shown="True" "Reset default" {
          frame False {
            # "True: Reset to default parameters\nFalse: Do nothing"
          }
          frame True {
            n201 = global read "GlobalInitialParamVals.vi" "InitialParamVals"() -> (w377:dbl[])
            n202 = call "GlobalParamAddress.vi"("Function select"="Read All") -> ("Parameter ID Out"=w380:dbl[])  [unwired: 3 in, 3 out]
            n203 = for {
              tunnel: w380 -> [w386] mode=indexing
              tunnel: w377 -> [w387] mode=indexing
              tunnel: [FALSE ("Wait")] -> w379
              tunnel: [w383] -> w376
              tunnel: w377 -> [w383]
              tunnel: [0.0 ("Page Select")] -> w375
              n204 = Wait (ms)(milliseconds to wait=u32 5) -> ()  [unwired: 1 out]
              n205 = call "GlobalTransmitBuffer7.vi"("Data_ID # in"=w386, "Value in"=w387, "Function select"="Write") -> ()  [unwired: 3 out]
            }
            n206 = local write "Page Select"(w375) -> ()
            n207 = local write "WAIT"(w379) -> ()
            n208 = local write "Input"(w376) -> ()
            "WAIT" <- TRUE ("Wait")
          }
        }
        n209 = Not Equal?(x=w251, y=w292) -> (x != y?=→"error":bool[])
      }
      frame "Data Select" {
        w484 = 24 ("length")
        w475 = 24 ("length")
        n210 = global read "GlobalDataSelectArray.vi" "Data Select Array"() -> (w471:bool[])
        n211 = Cluster To Array(cluster="?") -> (array=w497:bool[])
        n212 = Cluster To Array(cluster="Select") -> (array=w499:bool[])
        n213 = local read "Two1"() -> (w459:bool[])
        n214 = local read "Two2"() -> (w460:bool[])
        n215 = local read "One1"() -> (w457:bool[])
        n216 = local read "One2"() -> (w458:bool[])
        n217 = call "GlobalDataAddress.vi"("Function select"="Read All") -> ("Data ID Out"=w469:dbl[], "Data Names Out"=w491:string[])  [unwired: 3 in, 2 out]
        n218 = Build Array (concatenate)(w499, w497) -> (w470:bool[])
        n219 = Build Array (concatenate)(w457, w458) -> (w455:bool[])
        n220 = Build Array (concatenate)(w459, w460) -> (w456:bool[])
        n221 = local read "Speed Sel 2"() -> (w452:enum32{"Slow", "Medium", "Fast"}[])
        n222 = local read "Speed Sel"() -> (w451:enum32{"Slow", "Medium", "Fast"}[])
        n223 = global read "GlobalDisplayIndex.vi" "display address"() -> (w468:dbl[])
        n224 = global read "GlobalDisplayIndex.vi" "display canID"() -> (w467:dbl[])
        n225 = Or Array Elements(Boolean array=w470) -> (logical OR=w461:bool)
        n226 = Increment(x="Page") -> (x+1=w486:dbl)
        n227 = Boolean To (0,1)(Boolean=w471) -> (0, 1=w507:i16[])
        n228 = Multiply(x="Page", y=24 ("length")) -> (x*y=w489:dbl)
        n229 = Multiply(x="Page", y=w475) -> (x*y=w477:dbl)
        n230 = Multiply(x=w486, y=24.0) -> (x*y=w488:dbl)
        n231 = Add Array Elements(numeric array=w507) -> (sum=w480:i16)
        "Number\nSelected" <- w480
        n232 = Build Array (concatenate)(w451, w452) -> (w464:enum32{"Slow", "Medium", "Fast"}[])
        n233 = Array Subset(array=w491, index=w489, length=24) -> (→"Array":string[])
        n234 = Less?(x=w480, y=i16 48) -> (x < y?=w496:bool)
        n235 = Array Subset(array=w469, index=w477, length=w475) -> (→"Data #":dbl[])
        n236 = call "GlobalIOData7.vi"("Function select"="Read All") -> ("Array"=w478:cluster{"Time":u32, "Value":sgl}[])  [unwired: 4 in, 1 out]
        n237 = Array Subset(array=w491, index=w488, length=24) -> (→"Array 2":string[])
        n238 = case shown="True" w496 {
          tunnel: w461 -> [w603 w650]
          tunnel: w470 -> [_ _]
          tunnel: "Page" -> [w600 w647]
          tunnel: w471 -> [w604 w640]
          tunnel: w470 -> [w602 w649]
          tunnel: w469 -> [w599 w648]
          tunnel: w468 -> [w601 w646]
          tunnel: w467 -> [w598 w645]
          tunnel: [w594 w644] -> w466
          tunnel: [w595 w643] -> w465
          tunnel: w464 -> [w597 w642]
          tunnel: [w596 w641] -> w463
          tunnel: w456 -> [_ w638]
          tunnel: w455 -> [_ w639]
          frame False {
            n239 = case shown="True" w603 {
              tunnel: w602 -> [_ w616]
              tunnel: w599 -> [_ w626]
              tunnel: w600 -> [_ w613]
              tunnel: w601 -> [w608 w625]
              tunnel: w598 -> [w607 w624]
              tunnel: [w607 w623] -> w595
              tunnel: [w608 w622] -> w594
              tunnel: w597 -> [w606 w621]
              tunnel: [w606 w620] -> w596
              tunnel: w604 -> [w605 w611]
              tunnel: [w605 w610] -> _
              frame False {
                # "The outer case structure being FALSE  indicates that the maximum of 48 data channels\nhas been reached"
                # "TRUE: Something has been eitehr selected or deselected \nFALSE: do nothing"
              }
              frame True {
                w609 = FALSE ("new element/subarray")
                n240 = Search 1D Array(1D array=w616, element=TRUE, start index (0)=0) -> (index of element=w618:i32)
                n241 = Multiply(x=24.0, y=w613) -> (x*y=w614:dbl)
                n242 = Add(x=w618, y=w614) -> (x+y=w612:dbl)
                n243 = Replace Array Subset(array=w611, new element=w609, index=w612) -> (w610:bool[])
                n244 = case shown="False" w609 {
                  tunnel: w626 -> [_ _]
                  tunnel: w625 -> [w633 w637]
                  tunnel: w624 -> [w632 w636]
                  tunnel: [w628 w636] -> w623
                  tunnel: [w629 w637] -> w622
                  tunnel: w621 -> [w631 w635]
                  tunnel: [w627 w635] -> w620
                  tunnel: w612 -> [w634 _]
                  frame False {
                    n245 = Search 1D Array(1D array=w633, element=w634) -> (index of element=w630:i32)  [unwired: 1 in]
                    n246 = Delete From Array(array=w633, index=w630) -> (array with subset deleted=w629:dbl[])  [unwired: 1 in, 1 out]
                    n247 = Delete From Array(array=w632, index=w630) -> (array with subset deleted=w628:dbl[])  [unwired: 1 in, 1 out]
                    n248 = Delete From Array(array=w631, index=w630) -> (array with subset deleted=w627:enum32{"Slow", "Medium", "Fast"}[])  [unwired: 1 in, 1 out]
                  }
                  frame True {
                    # "True: do nothing (array is full)\nFalse: remove from data array"
                  }
                }
                n249 = global write "GlobalDataSelectArray.vi" "Data Select Array"(w610) -> ()
              }
            }
          }
          frame True {
            n250 = case shown="True" w650 {
              tunnel: w649 -> [_ w665]
              tunnel: w648 -> [_ w675]
              tunnel: w647 -> [_ w662]
              tunnel: w646 -> [w654 w674]
              tunnel: w645 -> [w653 w673]
              tunnel: [w653 w672] -> w643
              tunnel: [w654 w671] -> w644
              tunnel: w642 -> [w652 w670]
              tunnel: [w652 w669] -> w641
              tunnel: w640 -> [w651 w659]
              tunnel: [w651 w657] -> _
              tunnel: w639 -> [_ w656]
              tunnel: w638 -> [_ w655]
              frame False {
                # "The outer case structure being TRUE  indicates that less than 48 data channels\nhave been selected"
                # "TRUE: Something has been either selected or deselected \nFALSE: do nothing"
              }
              frame True {
                n251 = Search 1D Array(1D array=w665, element=TRUE, start index (0)=0) -> (index of element=w667:i32)
                n252 = Multiply(x=24.0, y=w662) -> (x*y=w663:dbl)
                n253 = Add(x=w667, y=w663) -> (x+y=w661:dbl)
                n254 = Index Array(array=w659, index=w661) -> (element=w660:bool)
                n255 = Not(x=w660) -> (.not. x?=w658:bool)
                n256 = Replace Array Subset(array=w659, new element=w658, index=w661) -> (w657:bool[])
                n257 = case shown="True" w658 {
                  tunnel: w675 -> [_ w702]
                  tunnel: w674 -> [w691 w701]
                  tunnel: w673 -> [w690 w699]
                  tunnel: [w687 w698] -> w672
                  tunnel: [w688 w697] -> w671
                  tunnel: w670 -> [w689 w696]
                  tunnel: [w686 w695] -> w669
                  tunnel: w661 -> [w692 w694]
                  tunnel: w656 -> [w685 _]
                  tunnel: w655 -> [w684 _]
                  frame False {
                    w681 = 24 ("index")
                    n258 = Search 1D Array(1D array=w691, element=w692) -> (index of element=w683:i32)  [unwired: 1 in]
                    n259 = Delete From Array(array=w684, index=w683) -> (array with subset deleted=w680:bool[])  [unwired: 1 in, 1 out]
                    n260 = Delete From Array(array=w685, index=w683) -> (array with subset deleted=w682:bool[])  [unwired: 1 in, 1 out]
                    n261 = Delete From Array(array=w691, index=w683) -> (array with subset deleted=w688:dbl[])  [unwired: 1 in, 1 out]
                    n262 = Delete From Array(array=w690, index=w683) -> (array with subset deleted=w687:dbl[])  [unwired: 1 in, 1 out]
                    n263 = Delete From Array(array=w689, index=w683) -> (array with subset deleted=w686:enum32{"Slow", "Medium", "Fast"}[])  [unwired: 1 in, 1 out]
                    n264 = Split 1D Array(array=w680, index=w681) -> (first subarray=w677:bool[], second subarray=w676:bool[])
                    n265 = Split 1D Array(array=w682, index=w681) -> (first subarray=w679:bool[], second subarray=w678:bool[])
                    n266 = local write "One1"(w679) -> ()
                    n267 = local write "Two1"(w677) -> ()
                    n268 = local write "One2"(w678) -> ()
                    n269 = local write "Two2"(w676) -> ()
                  }
                  frame True {
                    # "True: add to data array\nFalse: remove from data array"
                    n270 = Index Array(array=w702, index=w694) -> (element=w700:dbl)
                    n271 = Build Array (concatenate)(w699, w700) -> (w698:dbl[])
                    n272 = Build Array (concatenate)(w701, w694) -> (w697:dbl[])
                    n273 = Build Array (concatenate)(w696, enum32{"Slow", "Medium", "Fast"}."Slow" ("Radio Buttons 2")) -> (w695:enum32{"Slow", "Medium", "Fast"}[])
                  }
                }
                n274 = global write "GlobalDataSelectArray.vi" "Data Select Array"(w657) -> ()
              }
            }
          }
        }
        n275 = for {
          tunnel: w469 -> [w584] mode=indexing
          tunnel: w478 -> [w585]
          tunnel: [w582] -> w474 mode=indexing
          # "Read in Values"
          n276 = Index Array(array=w585, index=w584) -> (element=w583:cluster{"Time":u32, "Value":sgl})
          n277 = Unbundle(w583) -> ("Value"=w582:sgl)  [unwired: 1 out]
        }
        n278 = Increment(x="Page") -> (x+1=w483:dbl)
        n279 = Multiply(x=w483, y=w484) -> (x*y=w476:dbl)
        n280 = Add(x=24.0 ("y"), y=w489) -> (x+y=w504:dbl)
        n281 = Array Subset(array=w469, index=w476, length=w484) -> (→"Data # 2":dbl[])
        n282 = Array Subset(array=w471, index=w489, length=24) -> (→"Indicator":bool[])
        n283 = Array Subset(array=w474, index=w476, length=w475) -> (→"Value 2":sgl[])
        n284 = Array Subset(array=w471, index=w504, length=24) -> (→"Indicator 2":bool[])
        n285 = Array Subset(array=w474, index=w477, length=w475) -> (→"Value 1":sgl[])
        n286 = case shown="False" FALSE {
          frame False {
            # "NOT FUNCTIONING YET!!\n\n\nTrue: Load saved data configuration\nfalse: do nothing"
            # "Need to write to global data num\nneed to reinitialize plot data table"
          }
          frame True {
            (unwired) enum16{"read/write", "read-only", "write-only"}."read-only" ("access (0:read/write)")
            w530 = enum32{"Slow", "Medium", "Fast"}[] [enum."Slow", enum."Slow", enum."Slow", enum."Slow", enum."Slow", enum."Slow", enum."Slow", enum."Slow", enum."Slow", enum."Slow", enum."Slow", enum."Slow", enum."Slow", enum."Slow", enum."Slow", enum."Slow", enum."Slow", enum."Slow", enum."Slow", enum."Slow", enum."Slow", enum."Slow", enum."Slow", enum."Slow"] items=["Slow", "Medium", "Fast"] ("Speed Sel 2")
            n287 = global read "GlobalDataSelectArray.vi" "Data Select Array"() -> (w515:bool[])
            n288 = Array Size(array=w515) -> (size(s)=w514:i32)
            n289 = Open/Create/Replace File(prompt="Please Select Data Channel File", operation (0:open)=T8."open") -> (refnum out=w518:refnum<file>)  [unwired: 4 in, 2 out]
            n290 = Read from Text File(file (use dialog)=w518) -> (refnum out=w522:refnum<file>, text=w520:string)  [unwired: 3 in, 2 out]
            n291 = Read from Text File(file (use dialog)=w522) -> (refnum out=w526:refnum<file>, text=w524:string, error out=w527:errorcluster)  [unwired: 3 in, 1 out]
            n292 = Close File(refnum=w526, error in=w527) -> ()  [unwired: 2 out]
            n293 = Initialize Array(FALSE, w514) -> (w512:bool[])
            n294 = Spreadsheet String To Array(format string="%d", spreadsheet string=w524, array type (2D Dbl)=w530) -> (array=w529:enum32{"Slow", "Medium", "Fast"}[])  [unwired: 1 in]
            n295 = Spreadsheet String To Array(format string="%d", spreadsheet string=w520, array type (2D Dbl)=sgl[] []) -> (array=w516:sgl[])  [unwired: 1 in]
            n296 = for {
              tunnel: w516 -> [w535] mode=indexing
              shift-right: [w533] -> w511
              shift-left: w512 -> [w536]
              n297 = Replace Array Subset(array=w536, new element=TRUE, index=w535) -> (w533:bool[])
            }
            n298 = global write "GlobalDisplayIndex.vi" "display address"(w516) -> ()
            n299 = Split 1D Array(array=w529, index=24) -> (first subarray=w531:enum32{"Slow", "Medium", "Fast"}[], second subarray=w532:enum32{"Slow", "Medium", "Fast"}[])
            n300 = local write "Speed Sel 2"(w532) -> ()
            n301 = local write "Speed Sel"(w531) -> ()
            n302 = global write "GlobalDataSelectArray.vi" "Data Select Array"(w511) -> ()
          }
        }
        n303 = global write "GlobalDisplayIndex.vi" "display address"(w466) -> ()
        n304 = global write "GlobalDisplayIndex.vi" "display canID"(w465) -> ()
        n305 = Split 1D Array(array=w463, index=24) -> (first subarray=w454:enum32{"Slow", "Medium", "Fast"}[], second subarray=w453:enum32{"Slow", "Medium", "Fast"}[])
        n306 = local write "Speed Sel 2"(w453) -> ()
        n307 = local write "Speed Sel"(w454) -> ()
        n308 = case shown="True" "Search \nButton" {
          frame False {
            # "True: Initialize search and return all search hits\nFalse: do nothing"
          }
          frame True {
            n309 = call "GlobalDataAddress.vi"("Function select"="Read All") -> ("Data ID Out"=w563:dbl[], "Data Names Out"=w565:string[])  [unwired: 3 in, 2 out]
            n310 = Initialize Array(T9 {"Numeric"=0.0, "String"="", "ignore case? (F)"=FALSE} ("cluster")) -> (w562:T10)  [unwired: 1 in]
            n311 = for {
              tunnel: w565 -> [w572] mode=indexing
              tunnel: w563 -> [w570] mode=indexing
              tunnel: "Search" -> [w574]
              shift-right: [w568] -> w561
              shift-left: w562 -> [w567]
              # "Search each Name for given string"
              n312 = Search and Replace String(case sensitive?=TRUE ("ignore case? (F)"), input string=w572, search string=w574) -> (number of replacements=w573:i32)  [unwired: 5 in, 3 out]
              n313 = Greater Than 0?(x=w573) -> (x > 0?=w571:bool)
              n314 = case shown="True" w571 {
                tunnel: w572 -> [_ w580]
                tunnel: w570 -> [_ w581]
                tunnel: [w575 w578] -> w568
                tunnel: w567 -> [w575 w577]
                frame False {
                }
                frame True {
                  n315 = Bundle("Numeric"=w581, "String"=w580, "ignore case? (F)"=FALSE) -> (w579:T9)  [unwired: 1 in]
                  n316 = Build Array (concatenate)(w577, w579) -> (w578:T10)
                }
              }
            }
            "Results" <- w561
            n317 = Array Size(array=w561) -> (size(s)=→"# of Results":i32)
          }
        }
        n318 = case shown="False" "save data" {
          frame False {
            # "NOT FUNCTIONING YET!!\n\n\nTrue: save data configuration\nfalse: do nothing"
          }
          frame True {
            w548 = "DataChannels.txt" ("Default file name")
            # "Generate time stamp"
            n319 = local read "Speed Sel"() -> (w557:enum32{"Slow", "Medium", "Fast"}[])
            n320 = local read "Speed Sel 2"() -> (w556:enum32{"Slow", "Medium", "Fast"}[])
            n321 = global read "GlobalDisplayIndex.vi" "display address"() -> (w553:dbl[])
            n322 = String Length(string=w548) -> (length=w546:i32)
            n323 = Format Date/Time String(time format string (%c)="-%Y%m%d-%H%M%S") -> (date/time string=w552:string)  [unwired: 2 in]
            n324 = Build Array (concatenate)(w557, w556) -> (w554:enum32{"Slow", "Medium", "Fast"}[])
            n325 = Subtract(x=w546, y=4) -> (x-y=w550:i32)
            n326 = Replace Substring(2:0, 3:w550, 4:w552, 5:w548) -> (1:w547:string)  [unwired: 1 out]
            n327 = Array To Spreadsheet String(array=w553, 3:"%d") -> (spreadsheet string=w538:string)  [unwired: 1 in]
            n328 = Array To Spreadsheet String(array=w554, 3:"%d") -> (spreadsheet string=w558:string)  [unwired: 1 in]
            n329 = File Dialog(9:w547) -> (0:w545:errorcluster, 3:w543:path)  [unwired: 6 in, 2 out]
            n330 = Unbundle(w545) -> ()  [unwired: 3 out]
            n331 = Open/Create/Replace File(file path (use dialog)=w543, operation (0:open)=T8."create") -> (refnum out=w541:refnum<file>)  [unwired: 4 in, 2 out]
            n332 = Write to Text File(file (use dialog)=w541, text=w538) -> (refnum out=w540:refnum<file>)  [unwired: 2 in, 2 out]
            n333 = Write to Text File(file (use dialog)=w540, text=w558) -> (refnum out=w539:refnum<file>)  [unwired: 2 in, 2 out]
            n334 = Close File(refnum=w539) -> ()  [unwired: 1 in, 2 out]
          }
        }
        n335 = case shown="True" w461 {
          tunnel: w465 -> [_ w587]
          frame False {
            # "True: Update plot table if a data channel\nhas been selected or deselected.\n\nFalse: do nothing"
          }
          frame True {
            n336 = flat-sequence {
              tunnel: w587 -> [w588]
              tunnel: [w588] -> w586
              tunnel: w586 -> [w590]
              frame #0 {
                n337 = call "GlobalPlotDataIDTable7.vi"("Function select"="Initialize") -> ()  [unwired: 3 in, 1 out]
              }
              frame #1 {
                n338 = for {
                  tunnel: w590 -> [w591] mode=indexing
                  i -> [w592]
                  n339 = call "GlobalPlotDataIDTable7.vi"("IO Data ID in"=w591, "Plot channel in"=w592, "Function select"="Write") -> ()  [unwired: 1 in, 1 out]
                }
              }
            }
          }
        }
        n340 = call "GlobalDataNum7.vi"("Data  Numbers In"=w465, "Function select"="Write All") -> ()  [unwired: 2 in, 2 out]
      }
      frame "Display Data" {
        # "Note: in order to set the speed you must assign a value of:\n\nVALUE = SPEEDVAL + CAN_ID# \n\nto the appropriate labview speed channel corresponding to the position\nof the data in the data table  \n\nSPEEDVAL is: \n                     0 for slow\n             65536 for medium\n           131072 for fast"
        # "Indexing the output here might be a problem\nwhen we're feeding into two different arrays..."
        # "Speed \"Translator\": Input a 48-element vector of data speed numbers. This function\nevaluates whether each number corresponds to a high, med, or low speed data \nvalue by checking what range it falls into. (Select range via \"range selectors\") Returns \na 48-element vector of color values, each either red, green, or yellow"
        n341 = global read "GlobalSpeedUpdateTime.vi" "Previous speed update time"() -> (w709:dbl)
        n342 = global read "GlobalDisplayIndex.vi" "display address"() -> (w712:dbl[])
        n343 = Tick Count (ms)() -> (millisecond timer value=w706:u32)
        n344 = Subtract(x=w706, y=w709) -> (x-y=w707:dbl)
        n345 = call "GlobalIOData7.vi"("Function select"="Read All") -> ("Array"=w710:cluster{"Time":u32, "Value":sgl}[])  [unwired: 4 in, 1 out]
        n346 = Greater?(x=w707, y=2000.0) -> (0:w705:bool)
        n347 = call "GlobalDataNum7.vi"("Function select"="Read All") -> ("Data Numbers Out"=w721:dbl[])  [unwired: 3 in, 1 out]
        n348 = Build Array (concatenate)("Speed Sel", "Speed Sel 2") -> (w727:enum32{"Slow", "Medium", "Fast"}[])
        n349 = for {
          N: 48 -> [_]
          tunnel: [w740] -> w726 mode=indexing
          tunnel: w727 -> [w729] mode=indexing
          tunnel: [w738] -> w720 mode=indexing
          tunnel: w721 -> [w733] mode=indexing
          tunnel: [w734] -> w716 mode=indexing
          tunnel: w712 -> [w730] mode=indexing
          tunnel: w710 -> [w737]
          tunnel: w706 -> [w732]
          tunnel: w705 -> [w731]
          tunnel: [w731] -> _
          i -> [w735]
          # "Reads and sets the data speeds based on what range\nthe values fall into."
          n350 = case shown="True" w731 {
            tunnel: [w741 w767] -> w740
            tunnel: w735 -> [w743 w765]
            tunnel: w733 -> [_ w761]
            tunnel: w732 -> [_ w760]
            tunnel: w729 -> [_ w746]
            frame False {
              n351 = local read "Speed 3"() -> (w744:u32[])
              n352 = local read "Speed 2"() -> (w745:u32[])
              n353 = Build Array (concatenate)(w745, w744) -> (w742:u32[])
              n354 = Index Array(array=w742, index=w743) -> (element=w741:u32)
            }
            frame True {
              n355 = global read "GlobalLabVIEWStart.vi" "LabVIEW Speed Channels"() -> (w766:dbl[])
              n356 = global write "GlobalSpeedUpdateTime.vi" "Previous speed update time"(w760) -> ()
              n357 = case shown="\"Fast\"" w746 {
                tunnel: [0 65536 131072] -> w762
                frame "Slow", Default {
                }
                frame "Medium" {
                }
                frame "Fast" {
                }
              }
              n358 = Index Array(array=w766, index=w765) -> (element=w758:dbl)
              n359 = Add(x=w762, y=w761) -> (x+y=w763:dbl)
              n360 = call "GlobalTransmitBuffer7.vi"("Data_ID # in"=w758, "Value in"=w763, "Function select"="Write") -> ()  [unwired: 3 out]
              n361 = call "GlobalIOData7.vi"("Function select"="Read One", "IO Data ID"=w758) -> ("IO data out"=w757:cluster{"Time":u32, "Value":sgl})  [unwired: 3 in, 1 out]
              n362 = Unbundle(w757) -> ("Value"=w756:sgl)  [unwired: 1 out]
              n363 = Less?(x=w756, y=sgl 5000.0) -> (x < y?=w753:bool)
              n364 = Less?(x=w756, y=sgl 70000.0) -> (x < y?=w752:bool)
              n365 = Select(t=1, s=w753, f=2) -> (s? t:f=w751:i32)
              n366 = Select(t=w751, s=w752, f=3) -> (s? t:f=w750:i32)
              n367 = case shown="2" w750 {
                tunnel: [w771 w775 w779] -> w767
                frame 1, Default {
                  # "Slow\n(red)"
                  n368 = call <vilib>:"RGB to Color.vi"("B"=u8 0, "G"=u8 0, "R"=u8 255) -> ("Color"=w771:u32)
                }
                frame 2 {
                  # "Medium\n(yellow)"
                  n369 = call <vilib>:"RGB to Color.vi"("B"=u8 0, "G"=u8 255, "R"=u8 255) -> ("Color"=w775:u32)
                }
                frame 3 {
                  # "Fast\n(green)"
                  n370 = call <vilib>:"RGB to Color.vi"("B"=u8 0, "G"=u8 255, "R"=u8 0) -> ("Color"=w779:u32)
                }
              }
            }
          }
          n371 = Index Array(array=w737, index=w733) -> (element=w736:cluster{"Time":u32, "Value":sgl})
          n372 = Unbundle(w736) -> ("Value"=w734:sgl)  [unwired: 1 out]
          n373 = call "GlobalDataAddress.vi"("Element index"=w730, "Function select"="Read One") -> ("Data name"=w738:string)  [unwired: 2 in, 3 out]
        }
        n374 = Split 1D Array(array=w726, index=24) -> (first subarray=→"Speed 2":u32[], second subarray=→"Speed 3":u32[])
        n375 = Split 1D Array(array=w720, index=24) -> (first subarray=→"Data Names 1":string[], second subarray=→"Data Names 2":string[])
        n376 = Split 1D Array(array=w716, index=24) -> (first subarray=→"Data Value 1":sgl[], second subarray=→"Data Value 2":sgl[])
      }
      frame "SUGGESTIONS" {
      }
      frame "Errors" {
      }
    }
    n377 = global read "GlobalBatteryVoltageID.vi" "Batt Voltage ID"() -> (w64:dbl)
    n378 = call "GlobalIOData7.vi"("Function select"="Read One", "IO Data ID"=w64) -> ("IO data out"=w65:cluster{"Time":u32, "Value":sgl})  [unwired: 3 in, 1 out]
    n379 = Unbundle(w65) -> ("Value"=→"BATTERY VOLTAGE":sgl)  [unwired: 1 out]
    n380 = call "GlobalDataNum7.vi"("Function select"="Read All") -> ("Data Numbers Out"=w76:dbl[])  [unwired: 3 in, 1 out]
    n381 = Array Subset(array=w76, index=0, length=24) -> (→"Channel # 1":dbl[])
    n382 = Array Subset(array=w76, index=24, length=24) -> (→"Channel # 2":dbl[])
    n383 = Build Array (concatenate)("Two1", "Two2") -> (w78:bool[])
    n384 = Build Array (concatenate)("One1", "One2") -> (w77:bool[])
    n385 = case shown="True" "Graph\non" {
      tunnel: w76 -> [_ w145]
      tunnel: w78 -> [_ w146]
      frame False {
        # "This case structure deals with all the graphing for graph 2"
      }
      frame True {
        # "Output of Names"
        # "Output of Values"
        # "GRAPH 2"
        # "Local Index Selector"
        n386 = Initialize Array(0.0 ("element")) -> (w140:dbl[])  [unwired: 1 in]
        n387 = Initialize Array(0 ("index of element")) -> (w143:i32[])  [unwired: 1 in]
        n388 = while {
          tunnel: w146 -> [w174]
          shift-right: [w159] -> _
          shift-left: 0 ("index of element") -> [w161]
          tunnel: w145 -> [w168]
          shift-right: [w164] -> w149
          shift-left: w140 -> [w169]
          shift-right: [w156] -> w148
          shift-left: w140 -> [w157]
          shift-right: [w155] -> w147
          shift-left: w143 -> [w154]
          stop <- w162 stop-if-true
          n389 = global read "GlobalDisplayIndex.vi" "display address"() -> (w158:dbl[])
          n390 = Search 1D Array(1D array=w174, element=TRUE, start index (0)=w161) -> (index of element=w160:i32)
          n391 = Not Equal?(x=w160, y=-1.0) -> (x != y?=w170:bool)
          n392 = case shown="True" w170 {
            tunnel: w160 -> [_ w182]
            tunnel: w169 -> [w177 w187]
            tunnel: w168 -> [_ w188]
            tunnel: [w177 w186] -> w164
            tunnel: w158 -> [_ w179]
            tunnel: w157 -> [w176 w184]
            tunnel: [w176 w183] -> w156
            tunnel: [w175 w181] -> w155
            tunnel: w154 -> [w175 w180]
            frame False {
            }
            frame True {
              n393 = Index Array(array=w188, index=w182) -> (element=w185:dbl)
              n394 = Index Array(array=w179, index=w182) -> (element=w178:dbl)
              n395 = Build Array (concatenate)(w180, w182) -> (w181:i32[])
              n396 = Build Array (concatenate)(w187, w185) -> (w186:dbl[])
              n397 = Build Array (concatenate)(w184, w178) -> (w183:dbl[])
            }
          }
          n398 = Array Size(array=w164) -> (size(s)=w165:i32)
          n399 = Increment(x=w160) -> (x+1=w159:i32)
          n400 = Equal?(x=w160, y=-1.0) -> (x = y?=w167:bool)
          n401 = Equal?(x=4.0, y=w165) -> (x = y?=w163:bool)
          n402 = Or(x=w167, y=w163) -> (x .or. y?=w162:bool)
        }
        n403 = call "GlobalDataAddress.vi"("Function select"="Read All") -> ("Data Names Out"=w153:string[])  [unwired: 3 in, 3 out]
        n404 = for {
          tunnel: w153 -> [w194]
          tunnel: [w193] -> w151 mode=indexing
          tunnel: [w191] -> w152 mode=indexing
          tunnel: w149 -> [_] mode=indexing
          tunnel: w148 -> [w190] mode=indexing
          tunnel: w147 -> [w189] mode=indexing
          n405 = Index Array(array=w194, index=w190) -> (element=w193:string)
          n406 = call "GlobalPlotData7.vi"("Function select"="Read", "Data channel #"=w189) -> ("Single data plot cluster"=w191:cluster{"Array":u32[], "Array 2":sgl[]})  [unwired: 3 in]
        }
        "Graph Two" <- w152
        "graph2labels" <- w151
      }
    }
    n407 = case shown="True" "Graph\non" {
      tunnel: w76 -> [_ w205]
      tunnel: w77 -> [_ w204]
      frame False {
        # "This case structure deals with all the graphing for graph 1"
      }
      frame True {
        # "GRAPH 1"
        # "Output of Names"
        # "Output of Values"
        # "Local Index Selector"
        # "Global Index Selector"
        n408 = Initialize Array(0 ("index of element")) -> (w197:i32[])  [unwired: 1 in]
        n409 = Initialize Array(0.0 ("element")) -> (w200:dbl[])  [unwired: 1 in]
        n410 = while {
          tunnel: w204 -> [w229]
          shift-right: [w214] -> _
          shift-left: 0 ("index of element") -> [w216]
          tunnel: w205 -> [w223]
          shift-right: [w219] -> w206
          shift-left: w200 -> [w224]
          shift-right: [w211] -> w199
          shift-left: w200 -> [w212]
          shift-right: [w210] -> w195
          shift-left: w197 -> [w209]
          stop <- w217 stop-if-true
          n411 = global read "GlobalDisplayIndex.vi" "display address"() -> (w213:dbl[])
          n412 = Search 1D Array(1D array=w229, element=TRUE, start index (0)=w216) -> (index of element=w215:i32)
          n413 = Not Equal?(x=w215, y=-1.0) -> (x != y?=w225:bool)
          n414 = case shown="True" w225 {
            tunnel: w215 -> [_ w237]
            tunnel: w224 -> [w232 w242]
            tunnel: w223 -> [_ w243]
            tunnel: [w232 w241] -> w219
            tunnel: w213 -> [_ w234]
            tunnel: w212 -> [w231 w239]
            tunnel: [w231 w238] -> w211
            tunnel: [w230 w236] -> w210
            tunnel: w209 -> [w230 w235]
            frame False {
            }
            frame True {
              n415 = Index Array(array=w234, index=w237) -> (element=w233:dbl)
              n416 = Index Array(array=w243, index=w237) -> (element=w240:dbl)
              n417 = Build Array (concatenate)(w235, w237) -> (w236:i32[])
              n418 = Build Array (concatenate)(w239, w233) -> (w238:dbl[])
              n419 = Build Array (concatenate)(w242, w240) -> (w241:dbl[])
            }
          }
          n420 = Array Size(array=w219) -> (size(s)=w220:i32)
          n421 = Increment(x=w215) -> (x+1=w214:i32)
          n422 = Equal?(x=w215, y=-1.0) -> (x = y?=w222:bool)
          n423 = Equal?(x=4.0, y=w220) -> (x = y?=w218:bool)
          n424 = Or(x=w222, y=w218) -> (x .or. y?=w217:bool)
        }
        n425 = call "GlobalDataAddress.vi"("Function select"="Read All") -> ("Data Names Out"=w208:string[])  [unwired: 3 in, 3 out]
        n426 = for {
          tunnel: w208 -> [w248]
          tunnel: w199 -> [w249] mode=indexing
          tunnel: [w247] -> w203 mode=indexing
          tunnel: [w245] -> w207 mode=indexing
          tunnel: w206 -> [_] mode=indexing
          tunnel: w195 -> [w244] mode=indexing
          n427 = Index Array(array=w248, index=w249) -> (element=w247:string)
          n428 = call "GlobalPlotData7.vi"("Function select"="Read", "Data channel #"=w244) -> ("Single data plot cluster"=w245:cluster{"Array":u32[], "Array 2":sgl[]})  [unwired: 3 in]
        }
        "Graph One" <- w207
        "graph1labels" <- w203
      }
    }
    n429 = global read "GlobalPlotUpdateTime.vi" "Prev Time"() -> (w70:dbl)
    n430 = Tick Count (ms)() -> (millisecond timer value=w71:u32)
    n431 = call "ErrorHandlerREADALL.vi"() -> ("Small Error Cluster Out"=w61:T7)  [unwired: 10 in, 1 out]
    n432 = case shown="False" "Clear Errors" {
      frame False {
        # "True: reset error variables\nFalse: do nothing"
      }
      frame True {
        n433 = global write "GlobalErrorCluster.vi" "Medium Error Cluster"(T7 [] ("Medium Error Cluster")) -> ()
        n434 = global write "GlobalErrorCluster.vi" "Cluster Timestamps"(dbl[] [] ("Cluster Timestamps")) -> ()
      }
    }
    n435 = call "ErrorHandlerUpdate.vi"("Small Input Cluster"=w61) -> ("Unsorted Timestamps"=w60:dbl[], "Full Error Cluster"=w59:T7)  [unwired: 9 in]
    n436 = call "GlobalStop7.vi"("Function select"="Read") -> ("stop"=w91:bool)
    n437 = Subtract(x=w71, y=w70) -> (x-y=w69:dbl)
    n438 = Greater?(x=w69, y=2000.0) -> (0:w67:bool)
    n439 = call "ErrorClusterSort2.vi"("Unsorted Timestamps"=w60, "Unsorted Errors"=w59) -> ("Sorted Timestamps"=w58:dbl[], "Sorted Errors"=w57:T7)  [unwired: 7 in]
    n440 = global write "GlobalErrorCluster.vi" "Cluster Timestamps"(w58) -> ()
    n441 = global write "GlobalErrorCluster.vi" "Medium Error Cluster"(w57) -> ()
    n442 = case shown="True" w67 {
      selector: w67 -> [w97 w109]
      frame False {
        # "True: cycle to next error message every 2 seconds\nFalse: keep displaying current error message"
        n443 = local write "error message"(w97) -> ()
      }
      frame True {
        n444 = Tick Count (ms)() -> (millisecond timer value=w98:u32)
        n445 = global read "GlobalErrorIndex.vi" "Err Index"() -> (w103:dbl)
        n446 = global read "GlobalErrorCluster.vi" "Medium Error Cluster"() -> (w106:T7)
        n447 = Array Size(array=w106) -> (size(s)=w104:i32)
        n448 = Decrement(x=w104) -> (x-1=w102:i32)
        n449 = global write "GlobalPlotUpdateTime.vi" "Prev Time"(w98) -> ()
        n450 = Greater?(x=w103, y=w102) -> (0:w101:bool)
        n451 = Select(t=0.0, s=w101, f=w103) -> (s? t:f=w99:dbl)
        n452 = Increment(x=w99) -> (x+1=w100:dbl)
        n453 = Array Subset(array=w106, index=w99, length=1) -> (w114:T7)
        n454 = call "ErrorHandlerLabel.vi"("Sorted Errors"=w114) -> ("Error Cluster Out"=w112:T11)  [unwired: 10 in]
        n455 = Index Array(array=w112, index=0) -> (element=w110:T12)
        n456 = Unbundle(w110) -> ("Error Name"=→"Error Name 1":string, "Board Name"=→"Board Name 1":string)  [unwired: 4 out]
        n457 = global write "GlobalErrorIndex.vi" "Err Index"(w100) -> ()
        "error message" <- w109
      }
    }
    n458 = call "ErrorHandlerLabel.vi"("Sorted Errors"=w57) -> ("Error Cluster Out"=w56:T11)  [unwired: 10 in]
    n459 = Wait Until Next ms Multiple(millisecond multiple=100) -> ()  [unwired: 1 out]
    n460 = case shown="False" "Pause Button" {
      tunnel: w56 -> [w115 _]
      frame False {
        n461 = for {
          tunnel: [w126] -> w120 mode=indexing
          tunnel: [w125] -> w119 mode=indexing
          tunnel: [w124] -> w118 mode=indexing
          tunnel: [w123] -> w117 mode=indexing
          tunnel: [w121] -> w116 mode=indexing
          tunnel: w115 -> [w122] mode=indexing
          n462 = Unbundle(w122) -> ("Frequency"=w126:dbl, "Description"=w125:string, "Error Name"=w124:string, "Board Name"=w123:string, "Timestamp"=w121:dbl)  [unwired: 1 out]
        }
        "Error Description" <- w119
        "Board" <- w117
        "Error Name" <- w118
        "Freq." <- w120
        "Time" <- w116
      }
      frame True {
        # "True: pause screen\nFalse: update fields"
      }
    }
    n463 = case shown="True" "stop" {
      frame False {
      }
      frame True {
        n464 = call "GlobalStop7.vi"("Function select"="Set") -> ()  [unwired: 1 out]
      }
    }
  }
